vi "TDM_Abhishek_Barla_Hardware.vi"() -> ()   [LabVIEW 2013]
panel:
  out "Recevied Composite  4":dynamicdata(graph)
  out "Recevied Composite  3":dynamicdata(graph)
  out "Recevied Composite  2":dynamicdata(graph)
  out "Recevied Composite":dynamicdata(graph)
  out "Sine":dbl[](graph)
  out "Sawtooth":dbl[](graph)
  out "Square":dbl[](graph)
  out "Waveform Graph 3-Swatooth":dynamicdata(graph)
  out "Waveform Graph 2 - Square":dynamicdata(graph)
  out "Waveform Graph 1 - Sine":dynamicdata(graph)
  # "Virtual Instrumentation Lab - Midterm Project- Hardware - Abhishek Barla"
  # "Software Generated Signals"
  # "Hardware Generated Signals"
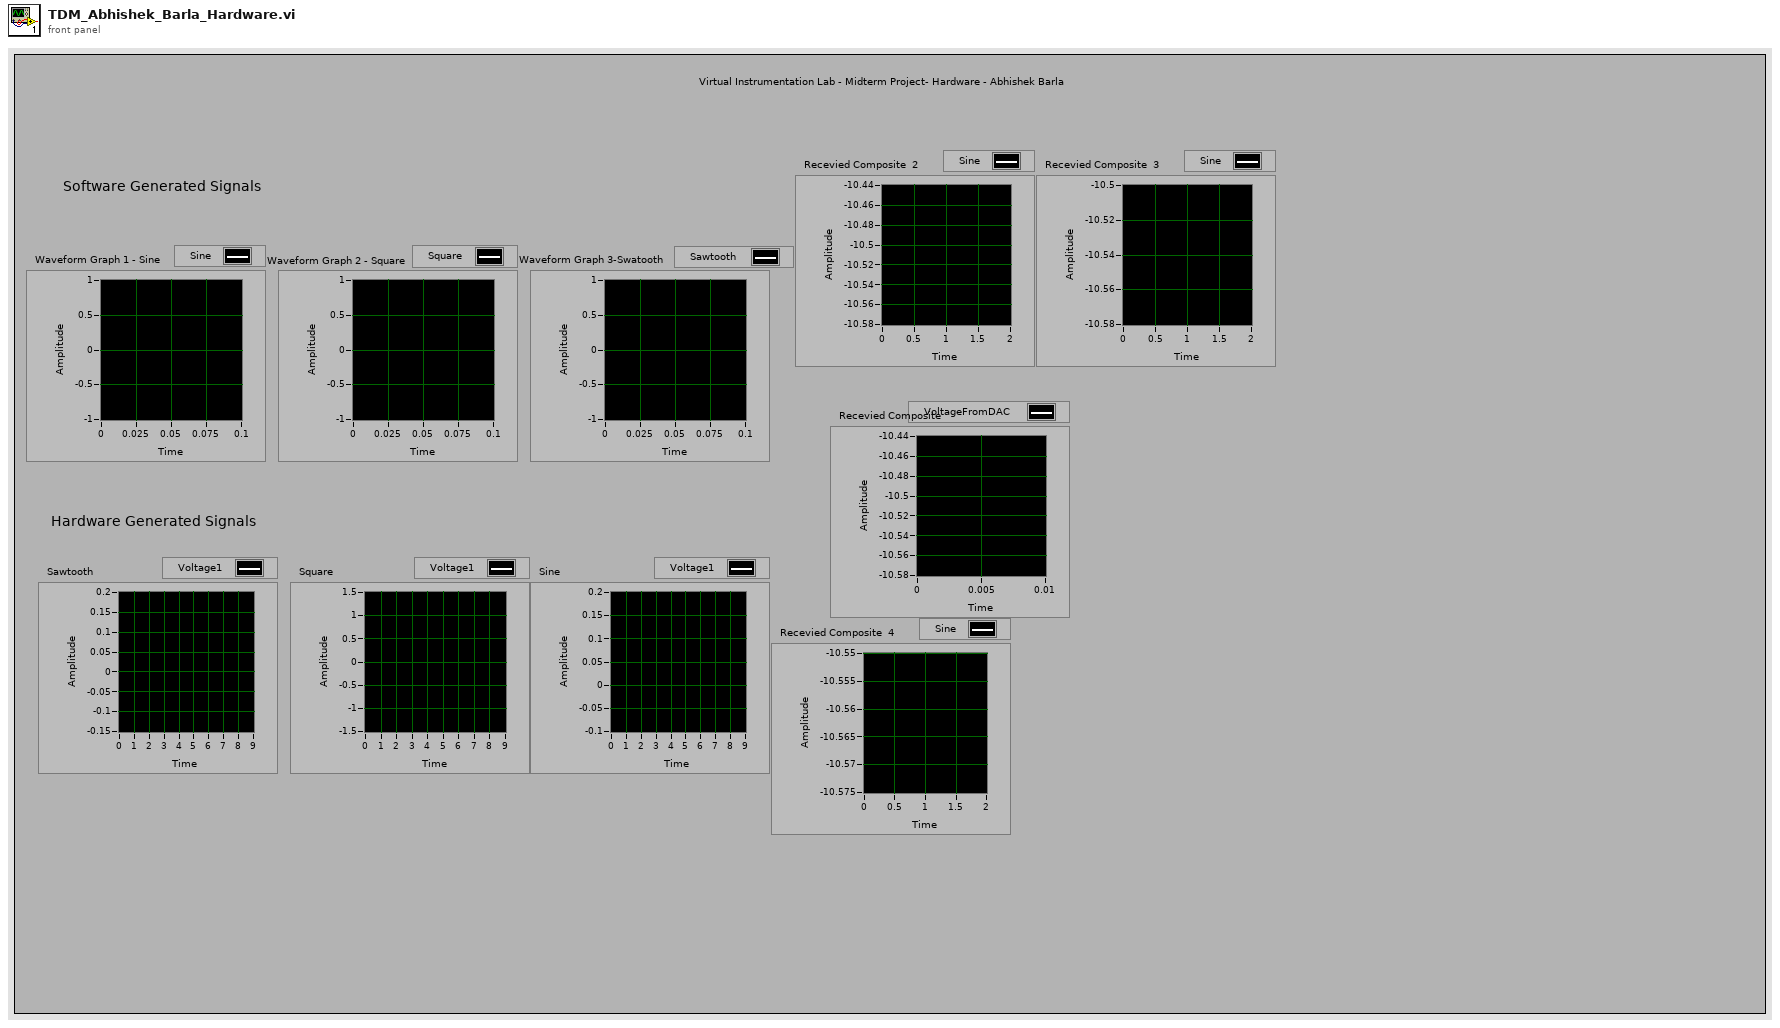
[diagram p1: front panel]
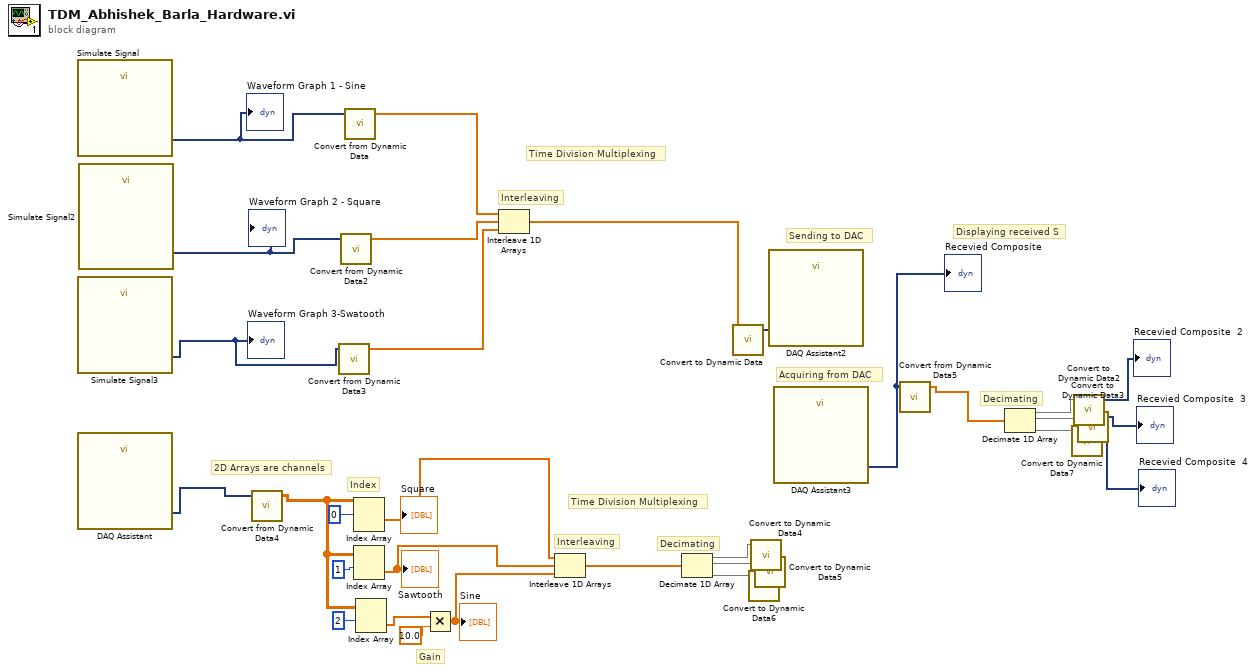
[diagram p0: block diagram]
diagram:
  # "Displaying received S"
  # "Decimating"
  # "Acquiring from DAC"
  # "Sending to DAC"
  # "Time Division Multiplexing"
  # "Time Division Multiplexing"
  # "Gain"
  # "Decimating"
  # "Interleaving"
  # "Index"
  # "2D Arrays are channels"
  # "Interleaving"
  n1 = call "Simulate Signal"() -> ("Sine"=w28:dynamicdata)  [unwired: 14 in, 1 out]
  "Waveform Graph 1 - Sine" <- w28
  n2 = call "Simulate Signal3"() -> ("Sawtooth"=w30:dynamicdata)  [unwired: 14 in, 1 out]
  "Waveform Graph 3-Swatooth" <- w30
  n3 = call "DAQ Assistant"() -> ("data"=w24:dynamicdata)  [unwired: 17 in, 2 out]
  n4 = call "Simulate Signal2"() -> ("Square"=w29:dynamicdata)  [unwired: 14 in, 1 out]
  "Waveform Graph 2 - Square" <- w29
  n5 = call "Convert from Dynamic Data4"("Dynamic Data Type"=w24) -> ("Array"=w21:dbl[][])  [unwired: 3 in]
  n6 = call "Convert from Dynamic Data3"("Dynamic Data Type"=w30) -> ("Array"=w25:dbl[])  [unwired: 3 in]
  n7 = call "Convert from Dynamic Data2"("Dynamic Data Type"=w29) -> ("Array"=w26:dbl[])  [unwired: 3 in]
  n8 = call "Convert from Dynamic Data"("Dynamic Data Type"=w28) -> ("Array"=w27:dbl[])  [unwired: 3 in]
  n9 = Index Array(array=w21, index (row)=0 ("index")) -> (element=w13:dbl[])  [unwired: 1 in]
  "Square" <- w13
  n10 = Index Array(array=w21, index (row)=1 ("index")) -> (element=w12:dbl[])  [unwired: 1 in]
  "Sawtooth" <- w12
  n11 = Index Array(array=w21, index (row)=2 ("index")) -> (element=w19:dbl[])  [unwired: 1 in]
  n12 = Multiply(x=w19, y=10.0) -> (x*y=w11:dbl[])
  "Sine" <- w11
  n13 = Interleave 1D Arrays(w27, w26, w25) -> (w10:dbl[])
  n14 = Interleave 1D Arrays(w13, w12, w11) -> (w17:dbl[])
  n15 = Decimate 1D Array(w17) -> (w16:dbl[], w15:dbl[], w14:dbl[])
  n16 = call "Convert to Dynamic Data"("Array"=w10) -> ("Dynamic Data Type"=w9:dynamicdata)  [unwired: 3 in]
  n17 = call "Convert to Dynamic Data6"("Array"=w14) -> ()  [unwired: 3 in, 1 out]
  n18 = call "Convert to Dynamic Data4"("Array"=w16) -> ()  [unwired: 3 in, 1 out]
  n19 = call "Convert to Dynamic Data5"("Array"=w15) -> ()  [unwired: 3 in, 1 out]
  n20 = call "DAQ Assistant2"("data"=w9) -> ()  [unwired: 17 in, 2 out]
  n21 = call "DAQ Assistant3"() -> ("data"=w4:dynamicdata)  [unwired: 17 in, 2 out]
  "Recevied Composite" <- w4
  n22 = call "Convert from Dynamic Data5"("Dynamic Data Type"=w4) -> ("Array"=w5:dbl[])  [unwired: 3 in]
  n23 = Decimate 1D Array(w5) -> (w8:dbl[], w7:dbl[], w6:dbl[])
  n24 = call "Convert to Dynamic Data7"("Array"=w6) -> ("Dynamic Data Type"=→"Recevied Composite  4":dynamicdata)  [unwired: 3 in]
  n25 = call "Convert to Dynamic Data2"("Array"=w8) -> ("Dynamic Data Type"=→"Recevied Composite  2":dynamicdata)  [unwired: 3 in]
  n26 = call "Convert to Dynamic Data3"("Array"=w7) -> ("Dynamic Data Type"=→"Recevied Composite  3":dynamicdata)  [unwired: 3 in]
